vi "SpeedIndicator.vi"(7 "ScaleUnit(F=km/h; T=knots)":bool, 8 "error in (no error)":errorcluster caption="Fehler (Eingang, kein Fehler)", 10 "MultiWii Data Cluster":T1 {"Altitude abs [m]" format="%.2f"; "Baro T [°C]" format="%.1f"; "Baro P [mbara]" format="%.1f"; "GPS_coord[LON]" format="%#_9f"; "GPS_coord[LAT]" format="%#_9f"; "Altitude [m]" format="%.2f"}) -> (0 "error out":errorcluster caption="Fehler (Ausgang)", 3 "SpeedIndicator":picture)   [LabVIEW 2017]
uses:
  IMU_Functions/IMU_Data_Cluster.ctl
  <vilib>/Utility/miscctls.llb/LVBoundsTypeDef.ctl
  <vilib>/picture/picture.llb/imagedata.ctl
panel:
  in  "Transparent":picture caption="Neue Grafik"
  # "switch control for speed unit\nF =km/h; T=knots"
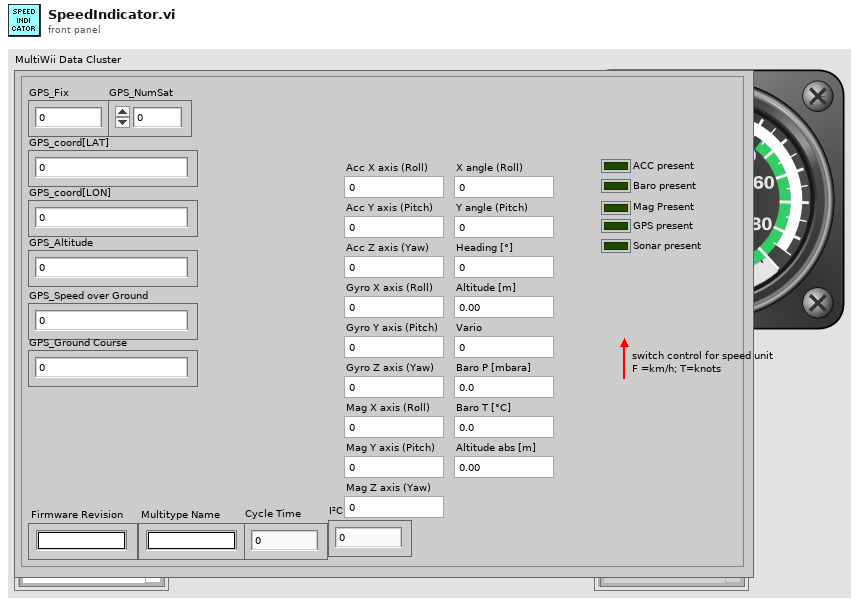
[diagram p1: front panel]
types:
  T1 = typedef "IMU_Data_Cluster.ctl" = cluster{"Firmware Revision":string, "Multitype Name":string, "Cycle Time":u16, "I²C Error Count":u16, "ACC present":bool, "Baro present":bool, "Mag Present":bool, "GPS present":bool, "Sonar present":bool, "Acc X axis (Roll)":dbl, "Acc Y axis (Pitch)":dbl, "Acc Z axis (Yaw)":dbl, "Gyro X axis (Roll)":dbl, "Gyro Y axis (Pitch)":dbl, "Gyro Z axis (Yaw)":dbl, "Mag X axis (Roll)":dbl, "Mag Y axis (Pitch)":dbl, "Mag Z axis (Yaw)":dbl, "X angle (Roll)":dbl, "Y angle (Pitch)":dbl, "Heading [°]":dbl, "Altitude [m]":dbl, "Vario":dbl, "GPS_Fix":u8, "GPS_NumSat":u8, "GPS_coord[LAT]":dbl, "GPS_coord[LON]":dbl, "GPS_Altitude":dbl, "GPS_Speed over Ground":dbl, "GPS_Ground Course":dbl, "Baro P [mbara]":dbl, "Baro T [°C]":dbl, "Altitude abs [m]":dbl}
  T2 = typedef "LVBoundsTypeDef.ctl" = cluster{"Width":u32, "Height":u32}
  T3 = typedef "imagedata.ctl" = cluster{"image type":i32, "image depth":i32, "image":u8[], "mask":u8[], "colors":u32[], "Rectangle":cluster{"left":i16, "top":i16, "right":i16, "bottom":i16}}
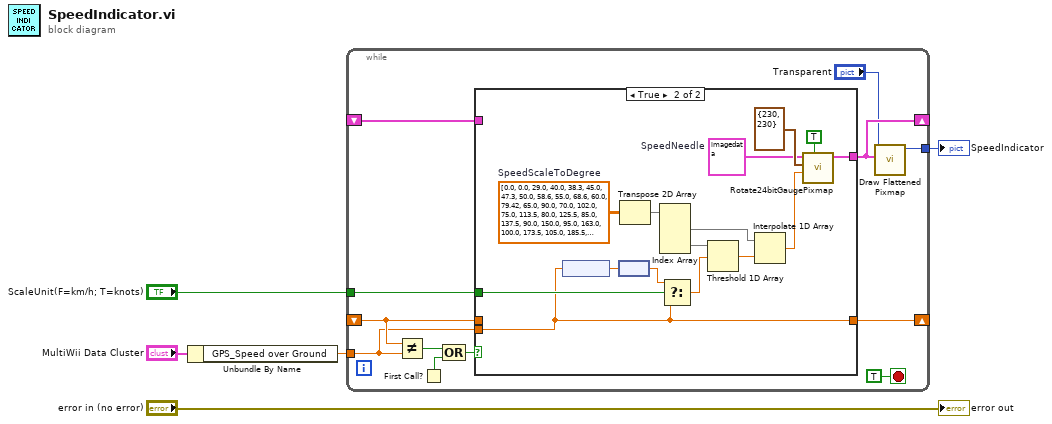
[diagram p0: block diagram]
diagram:
  n1 = Unbundle By Name("MultiWii Data Cluster") -> ("GPS_Speed over Ground"=w1:dbl)
  n2 = while {
    shift-right: [w14] -> _
    shift-left: _ -> [w13]
    tunnel: w1 -> [w8]
    shift-right: [w12] -> _
    shift-left: _ -> [w11]
    tunnel: [w9] -> w5
    tunnel: "ScaleUnit(F=km/h; T=knots)" -> [w7]
    stop <- TRUE stop-if-true
    n3 = Not Equal?(x=w13, y=w8) -> (x != y?=w15:bool)
    n4 = First Call?() -> (First Call?: T/F=w16:bool)
    n5 = Compound Arithmetic op=OR(w15, w16) -> (w17:bool)
    n6 = case shown="True" w17 {
      tunnel: [w19 w34] -> w12
      tunnel: w11 -> [w19 _]
      tunnel: w13 -> [w18 _]
      tunnel: [w18 w21] -> w14
      tunnel: w8 -> [_ w21]
      tunnel: w7 -> [_ w23]
      frame False {
      }
      frame True {
        w20 = T3 {"image type"=0, "image depth"=24, "image"=array[158700 elements], "mask"=[], "colors"=[], "Rectangle"={"left"=0, "top"=0, "right"=230, "bottom"=230}}  # SpeedNeedle
        w28 = dbl[][] [[0.0, 0.0], [29.0, 40.0], [38.3, 45.0], [47.3, 50.0], [58.6, 55.0], [68.6, 60.0], [79.42, 65.0], [90.0, 70.0], [102.0, 75.0], [113.5, 80.0], [125.5, 85.0], [137.5, 90.0], [150.0, 95.0], [163.0, 100.0], [173.5, 105.0], [185.5, 110.0], [196.5, 115.0], [207.3, 120.0], [215.2, 125.0], [224.0, 130.0], [231.8, 135.0], [239.8, 140.0], [247.3, 145.0], [254.3, 150.0], [261.7, 155.0], [268.7, 160.0], [273.7, 165.0], [281.0, 170.0], [286.7, 170.0], [286.8, 175.0], [292.8, 180.0], [299.4, 185.0], [305.8, 190.0], [311.8, 195.0], [318.0, 200.0]]  # SpeedScaleToDegree
        n7 = node(w21) -> (w30:dbl[unit])
        n8 = node(w30) -> (w31:dbl)
        n9 = Transpose 2D Array(2D array=w28) -> (transposed array=w25:dbl[][])
        n10 = Index Array(array=w25) -> (element #1=w27:dbl[], element #2=w26:dbl[])  [unwired: 4 in]
        n11 = Select(t=w31, s=w23, f=w21) -> (s? t:f=w29:dbl)
        n12 = Threshold 1D Array(2:w29, 3:w26) -> (0:w24:dbl)  [unwired: 1 in]
        n13 = Interpolate 1D Array(1:w24, 2:w27) -> (0:w22:dbl)
        n14 = call "Rotate24bitGaugePixmap.vi"("Maske kombinieren? (F)"=TRUE, "Rotation Angle (degrees)"=w22, "Größe des Darstellungsbereichs"=T2 {"Width"=230, "Height"=230}, "image data"=w20) -> ("image data out"=w34:T3)  [unwired: 7 in]
      }
    }
    n15 = call <vilib>:"Draw Flattened Pixmap.vi"("image data"=w12, "picture"="Transparent") -> ("new picture"=w9:picture)  [unwired: 7 out]
  }
  "SpeedIndicator" <- w5
  "error out" <- "error in (no error)"
